vi "CheckValidReference.vi"(8 "error in":errorcluster, 11 "message ref in":refnum<class "CLM_LocalMessage_Queue.lvclass">) -> (0 "error out":errorcluster, 2 "valid?":bool, 3 "message ref out":refnum<class "CLM_LocalMessage_Queue.lvclass">)   [LabVIEW 2013, in "CLM_LocalMessage_Queue.lvclass"]
uses:
  CLM_LocalMessage_Queue.lvclass
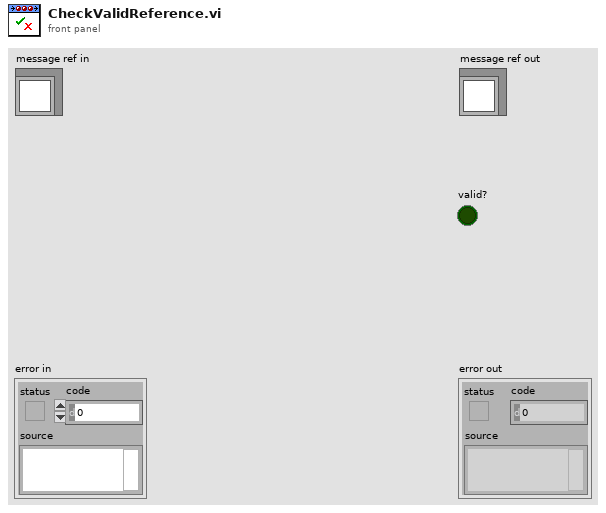
[diagram p1: front panel]
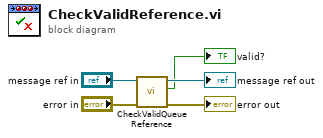
[diagram p0: block diagram]
diagram:
  n1 = call "CheckValidQueueReference.vi"("error in"="error in", "message ref in"="message ref in") -> ("error out"=→"error out":errorcluster, "valid?"=→"valid?":bool, "message ref out"=→"message ref out":refnum<class "CLM_LocalMessage_Queue.lvclass">)  [unwired: 7 in]
